vi "subSystem1.vi"() -> ()   [LabVIEW 2012, in "GUILib.lvlib"]
doc: "example of a sub-system"
uses:
  GUILib.lvlib
  GUILib.userEventsMainType.ctl
  UtilityLib/UtilityLib.valueStatus.ctl
  UtilityLib/UtilityLib.lvlib
panel:
  in  "stop":bool
  in  "subSystem1-4":bool
  in  "dummy":bool
  in  "parentSystem":bool
  in  "userEventsMain":T1
  in  "subSystem1-3":bool
  in  "userEvent":refnum<user-event>
  in  "subSystem1-2":bool
  in  "subSystem1-1":bool
  out "subSystem1-4state":bool
  out "subSystem1-3state":bool
  out "subSystem1-2state":bool
  out "subSystem1-1state":bool
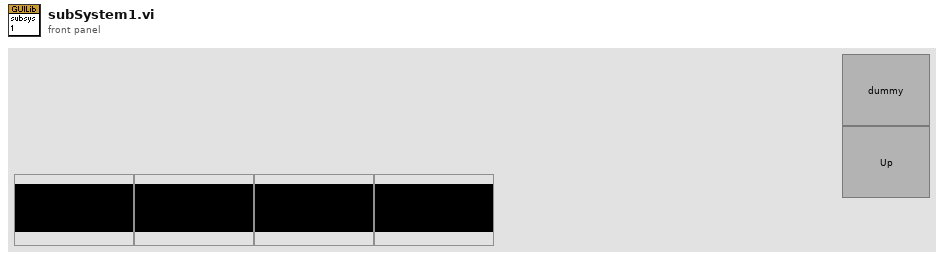
[diagram p1: front panel]
types:
  T1 = typedef "GUILib.lvlib/GUILib.userEventsMainType.ctl" = cluster{"data":string, "dataType":i32}
  T2 = typedef "UtilityLib.lvlib/UtilityLib.valueStatus.ctl" = enum16{"no info available", "stand by/off", "on", "warning", "alarm/malfunction", "not implemented", "user action required", "important information", "system default", "control default", "indicator default", "button default"}
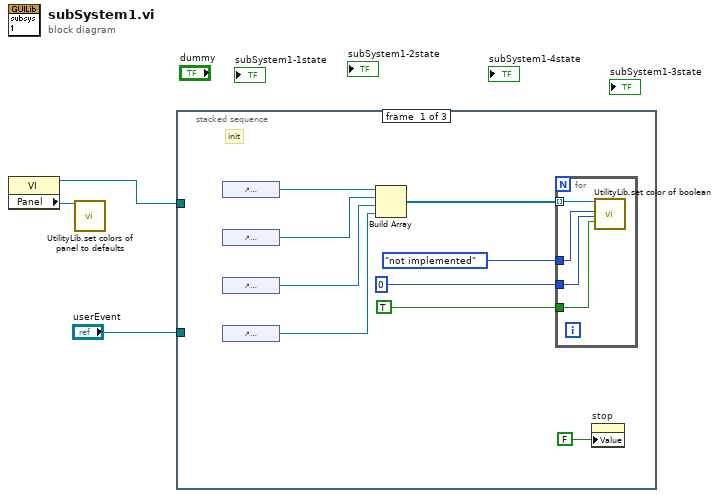
[diagram p0: block diagram]
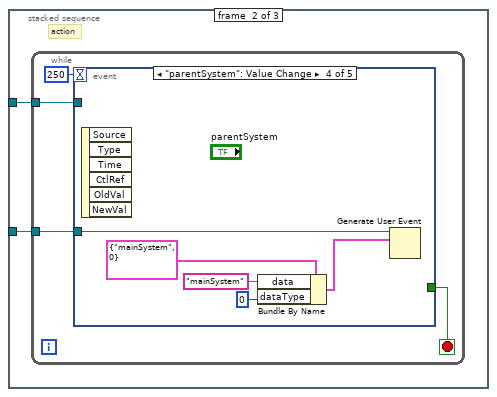
[diagram p2: hidden frame]
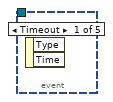
[diagram p3: hidden frame]
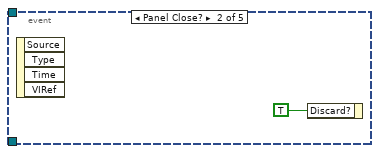
[diagram p4: hidden frame]
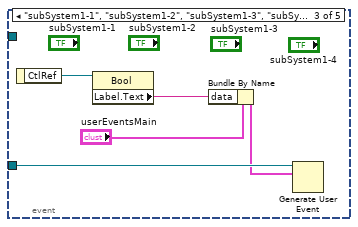
[diagram p5: hidden frame]
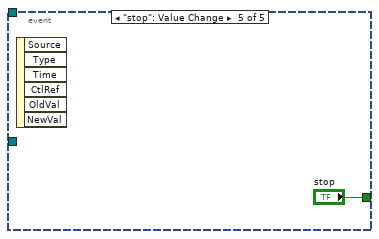
[diagram p6: hidden frame]
diagram:
  n1 = property on="Property Node" class="VI"() -> (reference out=w1:refnum<vi>, "Panel"=w2:refnum<vi>)  [unwired: 2 in, 1 out]
  n2 = call "UtilityLib.set colors of panel to defaults.vi"("Front Panel"=w2) -> ()  [unwired: 18 in, 1 out]
  n3 = stacked-sequence {
    tunnel: "userEvent" -> [_ w18 _]
    tunnel: w1 -> [_ w17 _]
    frame #0 {
      # "init"
      n4 = control-ref of="subSystem1-1state"() -> (w11:refnum<vi>)
      n5 = control-ref of="subSystem1-2state"() -> (w10:refnum<vi>)
      n6 = control-ref of="subSystem1-3state"() -> (w9:refnum<vi>)
      n7 = control-ref of="subSystem1-4state"() -> (w8:refnum<vi>)
      n8 = Build Array(w11, w10, w9, w8) -> (w4:refnum<vi>[])
      n9 = for {
        tunnel: UtilityLib.valueStatus."not implemented" ("valueStatus") -> [w16]
        tunnel: 0 ("nOfPair (0)") -> [w15]
        tunnel: TRUE ("setTRUEColor (FALSE)") -> [w14]
        tunnel: w4 -> [w13] mode=indexing
        n10 = call "UtilityLib.set color of boolean.vi"("button"=w13, "valueStatus"=w16, "nOfPair (0)"=w15, "setTRUEColor (FALSE)"=w14) -> ()  [unwired: 15 in, 1 out]
      }
      n11 = property on="stop" class="Bool (strict)"("Value"=FALSE ("stop")) -> ()  [unwired: 2 in, 2 out]
    }
    frame #1 {
      # "action"
      n12 = while {
        tunnel: w18 -> [w22]
        tunnel: w17 -> [w20]
        stop <- w19 stop-if-true
        n13 = event shown="[3] \"parentSystem\": Value Change" {
          selector: _ -> [_ _ _ _ _]
          dyn-events: _ -> [_ _ _ _ _]
          timeout: 250 -> [_ _ _ _ _]
          tunnel: w22 -> [_ _ w28 w33 _]
          tunnel: w20 -> [_ _ _ _ _]
          tunnel: [_ _ _ _ "stop"] -> w19
          event Timeout {
            n14 = event-data() -> ()  [unwired: 1 in, 2 out]
          }
          event Panel Close? {
            n15 = event-data() -> ()  [unwired: 1 in, 4 out]
            n16 = event-data ("Event Filter Node")("Discard?"=TRUE) -> ()  [unwired: 1 in, 1 out]
          }
          event "subSystem1-1", "subSystem1-2", "subSystem1-3", "subSystem1-4": Value Change {
            n17 = event-data() -> ("CtlRef"=w27:refnum<vi>)  [unwired: 1 in]
            n18 = property on="Property Node" class="Bool"(reference=w27) -> ("Label.Text"=w25:string)  [unwired: 1 in, 2 out]
            n19 = Bundle By Name(cluster="userEventsMain", "data"=w25) -> (w24:T1)
            n20 = Generate User Event(user event=w28, event data cluster=w24) -> ()  [unwired: 1 in, 2 out]
          }
          event "parentSystem": Value Change {
            n21 = event-data() -> ()  [unwired: 1 in, 6 out]
            n22 = Bundle By Name(cluster=T1 {"data"="mainSystem", "dataType"=0} ("userEventsMain"), "data"="mainSystem", "dataType"=0) -> (w31:T1)
            n23 = Generate User Event(user event=w33, event data cluster=w31) -> ()  [unwired: 1 in, 2 out]
          }
          event "stop": Value Change {
            n24 = event-data() -> ()  [unwired: 1 in, 6 out]
          }
        }
      }
    }
    frame #2 {
      # "deinit"
    }
  }
